vi "test1.vi"() -> ()   [LabVIEW 2021]
uses:
  <vilib>/ni845x/ni845x.llb/ni845xControl.ctl
  <vilib>/ni845x/ni845x.llb/NI-845x I2C Close Configuration Reference.vi
  <vilib>/ni845x/ni845x.llb/NI-845x Close Device Reference.vi
  <vilib>/ni845x/ni845x.llb/NI-845x I2C Slave Close Configuration Reference.vi
  <resource>/objmgr/NI845x.rc
panel:
  out "read data":u8[](array[numeric])
  in  "Write Delay Between Pages (ms)":u32=4
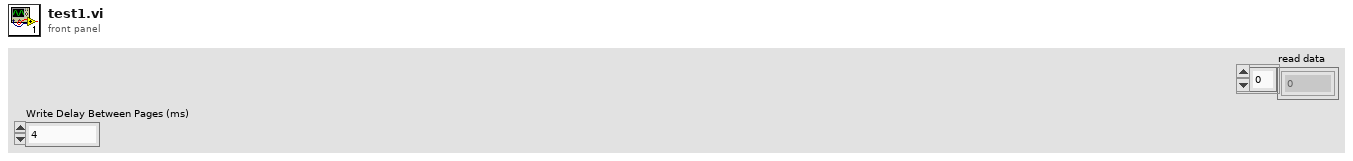
[diagram p1: front panel]
types:
  T1 = typedef "ni845xControl.ctl" = refnum<k21>
  T2 = typedef "ni845xI2cSlaveConfiguration.ctl" = refnum<k20>
  T3 = typedef "ni845xI2cConfiguration.ctl" = refnum<k20>
  T4 = typedef "ni845xI2cSlaveEventType.ctl" = enum8{"NoEvent", "CmdEvent", "DataAvailEvent", "DataReqEvent", "WriteCompleteEvent"}
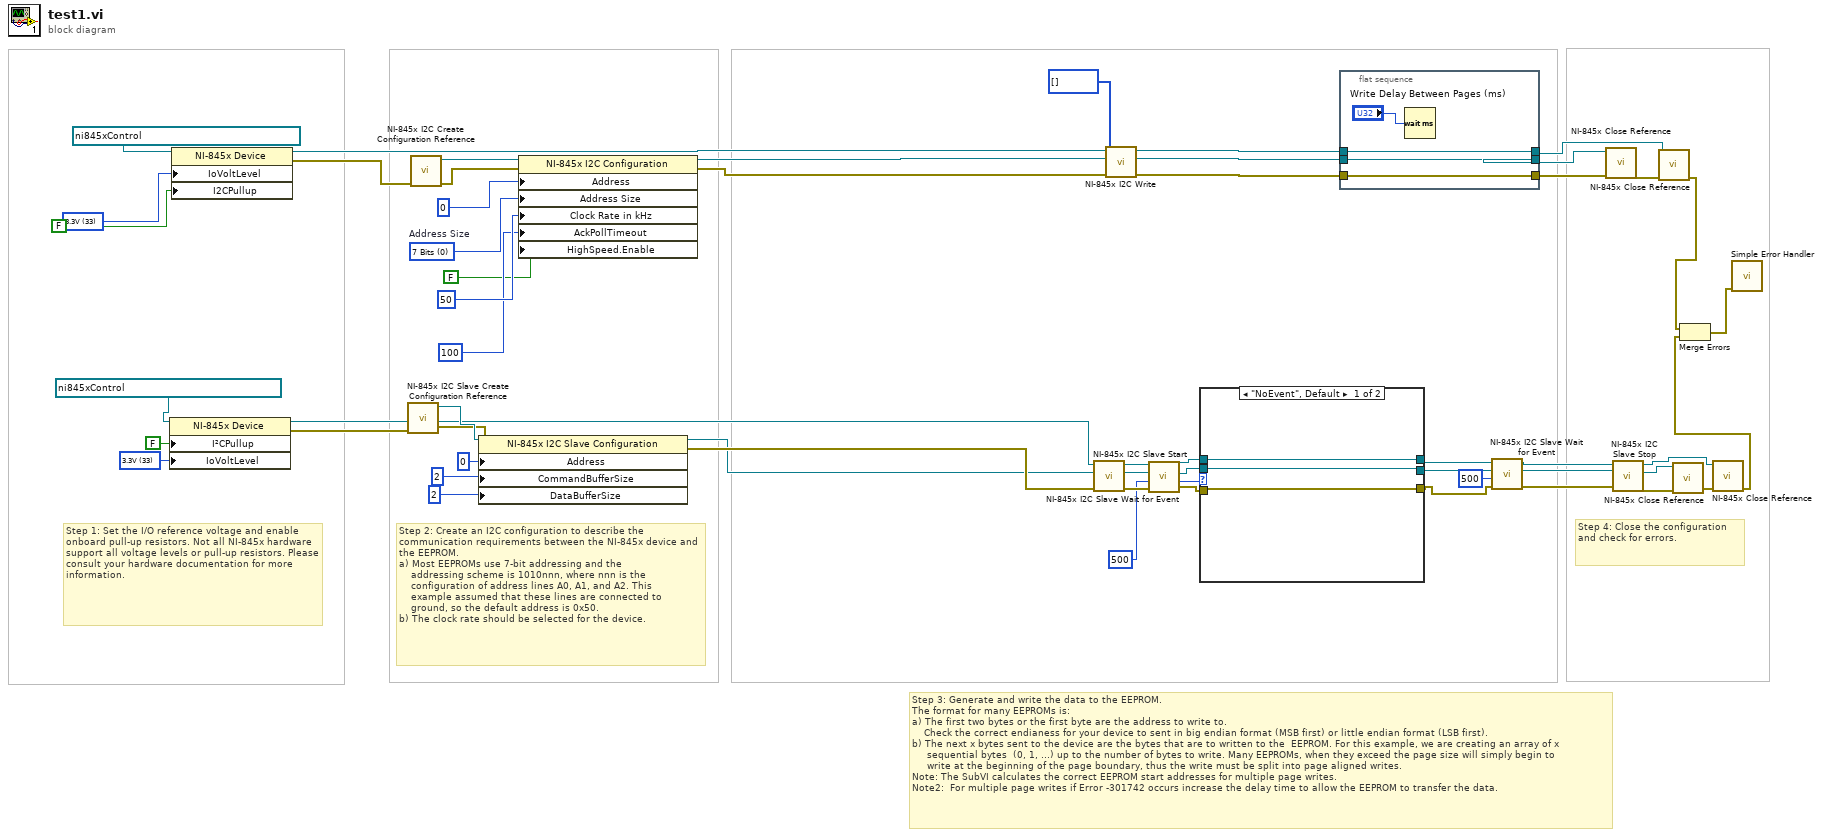
[diagram p0: block diagram]
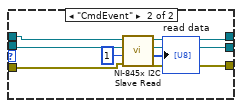
[diagram p2: hidden frame]
diagram:
  w38 = 33 items=["3.3V"=33, "2.5V"=25, "1.8V"=18, "1.5V"=15, "1.2V"=12] ("I/O Voltage Level")
  w44 = 33 items=["3.3V"=33, "2.5V"=25, "1.8V"=18, "1.5V"=15, "1.2V"=12] ("I/O Voltage Level")
  w55 = 0 items=["7 Bits", "10 Bits"]  # Address Size
  # "Step 1: Set the I/O reference voltage and enable onboard pull-up resistors. Not all NI-845x hardware support all voltage levels or pull-up resistors. Please consult your hardware documentation for more information."
  # "Step 4: Close the configuration \nand check for errors."
  # "Step 2: Create an I2C configuration to describe the \ncommunication requirements between the NI-845x device and the EEPROM.\na) Most EEPROMs use 7-bit addressing and the\n    addressing scheme is 1010nnn, where nnn is the\n    configuration of address lines A0, A1, and A2. This    \n    example assumed that these lines are connected to\n    ground, so the default address is 0x50. \nb) The clock rate should be selected for the device."
  # "Step 3: Generate and write the data to the EEPROM. \nThe format for many EEPROMs is:\na) The first two bytes or the first byte are the address to write to. \n    Check the correct endianess for your device to sent in big endian format (MSB first) or little endian format (LSB first).\nb) The next x bytes sent to the device are the bytes that are to written to the  EEPROM. For this example, we are creating an array of x\n     sequential bytes  (0, 1, ...) up to the number of bytes to write. Many EEPROMs, when they exceed the page size will simply begin to\n     write at the beginning of the page boundary, thus the write must be split into page aligned writes.\nNote: The SubVI calculates the correct EEPROM start addresses for multiple page writes.\nNote2:  For multiple page writes if Error -301742 occurs increase the delay time to allow the EEPROM to transfer the data."
  n1 = property class="NI-845x Device"(reference=T1 "USB0::0x3923::0x7514::01B67097::RAW" ("device reference"), "I²CPullup"=FALSE ("I²C Pullup Enable"), "IoVoltLevel"=w38) -> (reference out=w32:T1, error out=w35:errorcluster)  [unwired: 1 in]
  n2 = property on="Property Node" class="NI-845x Device"(reference=T1 "USB0::0x3923::0x7166::01B0380C::RAW" ("Device"), "IoVoltLevel"=w44, "I2CPullup"=FALSE ("Use Internal I2C Pullup Resistor")) -> (reference out=w46:T1, error out=w45:errorcluster)  [unwired: 1 in]
  n3 = call <vilib>:"NI-845x I2C Slave Create Configuration Reference.vi"("error in (no error)"=w35) -> ("error out"=w36:errorcluster, "i2c slave configuration"=w37:T2)  [unwired: 9 in]
  n4 = call <vilib>:"NI-845x I2C Create Configuration Reference.vi"("error in (no error)"=w45) -> ("error out"=w52:errorcluster, "i2c configuration"=w53:T3)  [unwired: 9 out]
  n5 = property class="NI-845x I2C Slave Configuration"(reference=w37, error in=w36, "Address"=u16 0, "CommandBufferSize"=u16 2, "DataBufferSize"=u16 2) -> (reference out=w18:T2, error out=w31:errorcluster)
  n6 = property on="Property Node" class="NI-845x I2C Configuration"(reference=w53, error in=w52, "Address"=u16 0, "Address Size"=w55, "Clock Rate in kHz"=u16 50 ("Clock Rate (kHz)"), "AckPollTimeout"=u16 100 ("ACK Poll Timeout"), "HighSpeed.Enable"=FALSE ("High Speed:Enable")) -> (reference out=w50:T3, error out=w49:errorcluster)
  n7 = call <vilib>:"NI-845x I2C Slave Start.vi"("error in (no error)"=w31, "i2c slave configuration in"=w18, "device reference in"=w32) -> ("error out"=w30:errorcluster, "i2c slave configuration out"=w19:T2, "device reference out"=w33:T1)  [unwired: 6 in]
  n8 = call <vilib>:"NI-845x I2C Write.vi"("error in (no error)"=w49, "write data"=u8[] [], "i2c configuration in"=w50, "device reference in"=w46) -> ("error out"=w27:errorcluster, "i2c configuration out"=w25:T3, "device reference out"=w26:T1)  [unwired: 5 in]
  n9 = call <vilib>:"NI-845x I2C Slave Wait for Event.vi"("error in (no error)"=w30, "timeout in ms (500)"=u32 500, "i2c slave configuration in"=w19, "device reference in"=w33) -> ("error out"=w22:errorcluster, "event type"=w21:T4, "i2c slave configuration out"=w24:T2, "device reference out"=w23:T1)  [unwired: 3 in, 1 out]
  n10 = case shown="\"NoEvent\", Default" w21 {
    tunnel: w24 -> [w58 w65]
    tunnel: w23 -> [w57 w67]
    tunnel: w22 -> [w59 w66]
    tunnel: [w59 w64] -> w4
    tunnel: [w58 w63] -> w6
    tunnel: [w57 w62] -> w7
    frame "NoEvent", Default {
    }
    frame "CmdEvent" {
      n11 = call <vilib>:"NI-845x I2C Slave Read.vi"("error in (no error)"=w66, "num bytes to read"=u16 1, "i2c slave configuration in"=w65, "device reference in"=w67) -> ("error out"=w64:errorcluster, "read data"=→"read data":u8[], "i2c slave configuration out"=w63:T2, "device reference out"=w62:T1)  [unwired: 3 in, 1 out]
    }
  }
  n12 = flat-sequence {
    tunnel: [w71] -> w51
    tunnel: [w70] -> w12
    tunnel: w26 -> [w70]
    tunnel: w27 -> [w71]
    tunnel: w25 -> [w69]
    tunnel: [w69] -> w48
    frame #0 {
      n13 = Wait (ms)(milliseconds to wait="Write Delay Between Pages (ms)") -> ()  [unwired: 1 out]
    }
  }
  n14 = call <vilib>:"NI-845x I2C Slave Wait for Event.vi"("error in (no error)"=w4, "timeout in ms (500)"=u32 500, "i2c slave configuration in"=w6, "device reference in"=w7) -> ("error out"=w3:errorcluster, "i2c slave configuration out"=w1:T2, "device reference out"=w2:T1)  [unwired: 3 in, 2 out]
  n15 = call-poly <vilib>:"NI-845x Close Reference.vi"("error in (no error)"=w51, "i2c configuration"=w48) -> ("error out"=w13:errorcluster)  [unwired: 9 out]
  n16 = call <vilib>:"NI-845x I2C Slave Stop.vi"("error in (no error)"=w3, "i2c slave configuration in"=w1, "device reference in"=w2) -> ("error out"=w16:errorcluster, "i2c slave configuration out"=w15:T2, "device reference out"=w8:T1)  [unwired: 6 in]
  n17 = call-poly <vilib>:"NI-845x Close Reference.vi"("error in (no error)"=w13, "device reference"=w12) -> ("error out"=w11:errorcluster)  [unwired: 9 out]
  n18 = call-poly <vilib>:"NI-845x Close Reference.vi"("error in (no error)"=w16, "i2c slave configuration"=w15) -> ("error out"=w9:errorcluster)  [unwired: 9 out]
  n19 = call-poly <vilib>:"NI-845x Close Reference.vi"("error in (no error)"=w9, "device reference"=w8) -> ("error out"=w10:errorcluster)  [unwired: 9 out]
  n20 = Merge Errors(w11, w10) -> (w17:errorcluster)
  n21 = call <vilib>:"Simple Error Handler.vi"("error in (no error)"=w17) -> ()  [unwired: 1 in, 8 out]
